vi "Check Variables & Linked Channels Correspondence.vi"(7 "Command/Response Refnum in":T1 format="%.0x", 8 "error in (no error)":errorcluster, 9 "Variables in":string[](array[string]), 11 "Linked Channels in":cluster{"Variable Name":string, "GUID":string}[](array[cluster])) -> (0 "error out":errorcluster, 3 "Linked Channels out":T2[](array[typedef]))   [LabVIEW 2020, in "Instrument Addon Scripting API.lvlib"]
uses:
  Instrument Addon Scripting API.lvlib
  Addon/Addon Shared/Types/Linked Channel Cluster.ctl
  <vilib>/NI VeriStand/Custom Device API/Custom Device Item Ref.ctl
  Addon/Addon Shared/Instrument Addon Shared.lvlib
  <vilib>/NI VeriStand/Custom Device API/Custom Device API.lvlib
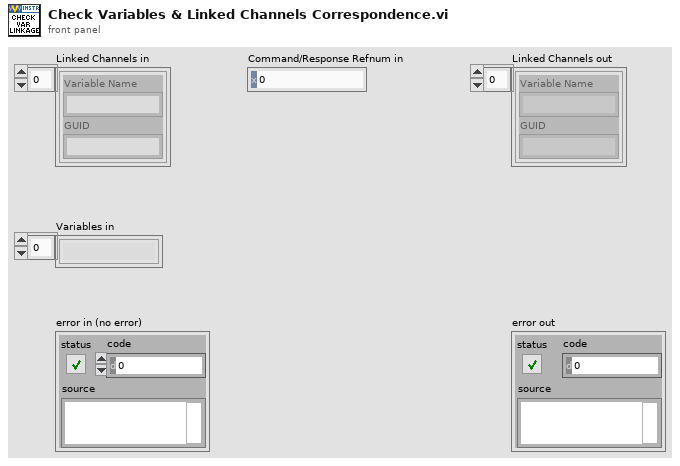
[diagram p1: front panel]
types:
  T1 = typedef "Custom Device API.lvlib/Custom Device Item Ref.ctl" = u64
  T2 = typedef "Instrument Addon Shared.lvlib/Linked Channel Cluster.ctl" = cluster{"Variable Name":string, "GUID":string}
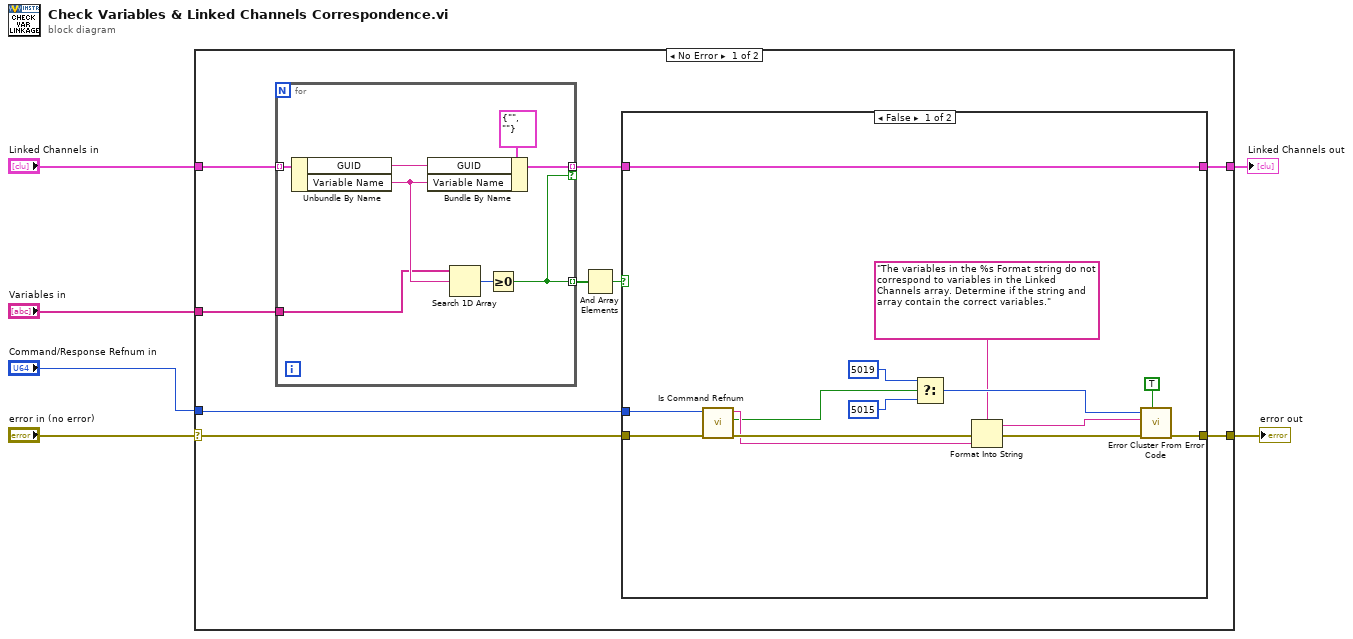
[diagram p0: block diagram]
diagram:
  n1 = case shown="No Error" "error in (no error)" {
    selector: "error in (no error)" -> [w8 w40]
    tunnel: "Linked Channels in" -> [w15 w41]
    tunnel: [w12 w40] -> w2
    tunnel: [w10 w41] -> w3
    tunnel: "Variables in" -> [w9 _]
    tunnel: "Command/Response Refnum in" -> [w7 _]
    frame No Error {
      n2 = for {
        tunnel: w15 -> [w38] mode=indexing
        tunnel: [w36] -> w11 mode=indexing if=w33
        tunnel: [w33] -> w14 mode=indexing
        tunnel: w9 -> [w32]
        n3 = Unbundle By Name(w38) -> ("GUID"=w37:string, "Variable Name"=w34:string)
        n4 = Bundle By Name(cluster=T2 {"Variable Name"="", "GUID"=""} ("Linked Channel"), "GUID"=w37, "Variable Name"=w34) -> (w36:T2)
        n5 = Search 1D Array(1D array=w32, element=w34) -> (index of element=w35:i32)  [unwired: 1 in]
        n6 = Greater Or Equal To 0?(x=w35) -> (x >= 0?=w33:bool)
      }
      n7 = And Array Elements(Boolean array=w14) -> (logical AND=w13:bool)
      n8 = case shown="False" w13 {
        tunnel: [w29 w30] -> w12
        tunnel: w11 -> [w28 w31]
        tunnel: [w28 w31] -> w10
        tunnel: w8 -> [w21 w30]
        tunnel: w7 -> [w20 _]
        frame False {
          n9 = call "Is Command Refnum.vi"("error in (no error)"=w21, "Command/Response Refnum in"=w20) -> ("error out"=w19:errorcluster, "Is Command?"=w17:bool, "Command/Response out"=w18:string)  [unwired: 7 in]
          n10 = Select(t=5019 ("error code (0)"), s=w17, f=5015 ("error code (0)")) -> (s? t:f=w24:i32)
          n11 = Format Into String(format string="The variables in the %s Format string do not correspond to variables in the Linked Channels array. Determine if the string and array contain the correct variables." ("error message (\"\")"), error in=w19, w18) -> (resulting string=w22:string, error out=w25:errorcluster)  [unwired: 1 in]
          n12 = call <vilib>:"Error Cluster From Error Code.vi"("show call chain? (False)"=TRUE, "error in (no error)"=w25, "error message (\"\")"=w22, "error code (0)"=w24) -> ("error out"=w29:errorcluster)  [unwired: 5 in]
        }
        frame True {
        }
      }
    }
    frame Error {
    }
  }
  "Linked Channels out" <- w3
  "error out" <- w2
